vi "GT Arc YZC Override2WN.vi"(0 "cardNum":i16, 1 "crd":i16, 2 "y":i32, 3 "z":i32, 4 "yCenter":dbl, 5 "zCenter":dbl, 6 "circleDir":i16, 7 "error in (no error)":errorcluster caption="错误输入（无错误）", 8 "synVel":dbl, 9 "synAcc":dbl, 10 "velEnd":dbl, 11 "segNum":i32, 12 "fifo":i16) -> (20 "function return":i16, 27 "error out":errorcluster caption="错误输出")   [LabVIEW 2020, in "gts.lvlib"]
doc: "GT_API GT_ArcYZCOverride2WN(short cardNum,short crd,long y,long z,double yCenter,double zCenter,short circleDir,double synVel,double synAcc,double velEnd=0,long segNum=0,short fifo=0);"
uses:
  gts.lvlib
  dll/32bit/multi_card/gts.dll
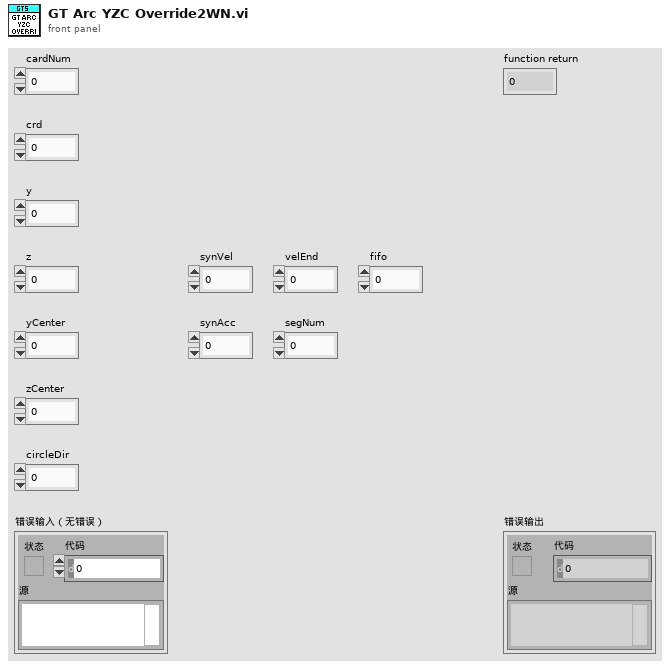
[diagram p1: front panel]
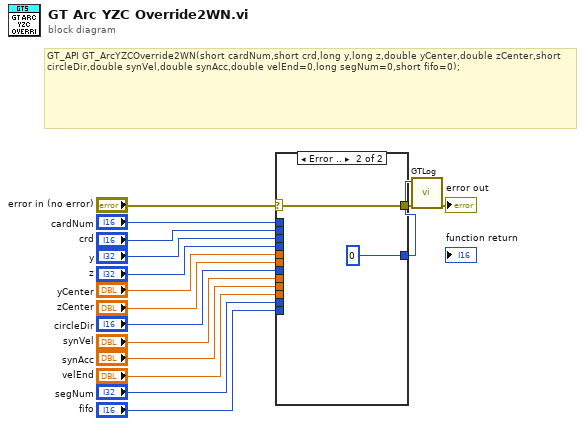
[diagram p0: block diagram]
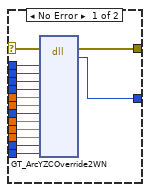
[diagram p2: hidden frame]
diagram:
  # "GT_API GT_ArcYZCOverride2WN(short cardNum,short crd,long y,long z,double yCenter,double zCenter,short circleDir,double synVel,double synAcc,double velEnd=0,long segNum=0,short fifo=0);"
  n1 = case shown="Error .." "error in (no error)" {
    selector: "error in (no error)" -> [w18 w33]
    tunnel: [w31 i16 0] -> w1
    tunnel: "cardNum" -> [w30 _]
    tunnel: "crd" -> [w29 _]
    tunnel: "y" -> [w28 _]
    tunnel: "z" -> [w27 _]
    tunnel: "yCenter" -> [w26 _]
    tunnel: "zCenter" -> [w25 _]
    tunnel: "circleDir" -> [w24 _]
    tunnel: "synVel" -> [w23 _]
    tunnel: "synAcc" -> [w22 _]
    tunnel: "velEnd" -> [w21 _]
    tunnel: "segNum" -> [w20 _]
    tunnel: "fifo" -> [w19 _]
    tunnel: [w17 w33] -> w3
    frame No Error {
      n2 = dll-call lib="C:/1228/dll/32bit/multi_card/gts.*" fn="GT_ArcYZCOverride2WN"(error in=w18, "cardNum"=w30, "crd"=w29, "y"=w28, "z"=w27, "yCenter"=w26, "zCenter"=w25, "circleDir"=w24, "synVel"=w23, "synAcc"=w22, "velEnd"=w21, "segNum"=w20, "fifo"=w19) -> (error out=w17:errorcluster, w31:i16)  [unwired: 14 in, 1 out]
    }
    frame Error {
    }
  }
  n3 = call "GTLog.vi"("error in (no error)"=w3, "Numeric"=w1) -> ("error out"=→"error out":errorcluster)  [unwired: 9 in]
